vi "Set Exp Time.vi"(0 "Notifier Name":string, 7 "Exp Time (s)":dbl, 11 "Error In":errorcluster) -> (4 "Notifier Name DUP":string, 6 "Running?":bool, 10 "Image Ref":T1, 15 "Error Out":errorcluster)   [LabVIEW 2020]
uses:
  <vilib>/vision/Image Controls.llb/IMAQ Image.ctl
  Hardware Configuration/Hardware Configuration Controls/Company.ctl
  Hamamatsu/Orca Flash/Orca Flash Controls/Orca Flash Parameters.ctl
  Hamamatsu/Orca Flash/Orca Flash Controls/Orca Flash Parameter List.ctl
  Hamamatsu/Orca Flash/Orca Flash Controls/Orca Flash Actions.ctl
  IDS/IDS Controls/IDS Actions.ctl
  IDS/IDS Controls/IDS Parameters.ctl
  IDS/IDS Controls/IDS Parameter List.ctl
  Photometrics/Prime BSI/R Cubed SITK/Prime BSI R3 Controls/Prime R3 Actions.ctl
  Photometrics/Prime BSI/R Cubed SITK/Prime BSI R3 Controls/Prime R3 Parameters.ctl
  Photometrics/Prime BSI/R Cubed SITK/Prime BSI R3 Controls/Prime R3 Parameter List.ctl
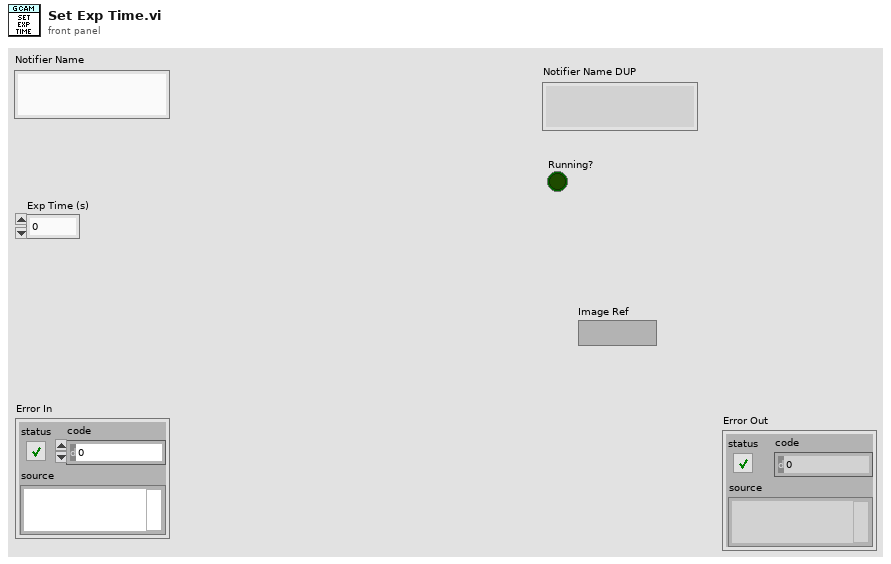
[diagram p1: front panel]
types:
  T1 = typedef "IMAQ Image.ctl" = refnum<image>
  T2 = typedef "Company.ctl" = enum16{"AA Opto Electronic", "ASI", "Coherent", "Creset Optics", "CVI", "DAQmx", "Hamamatsu", "IDS", "Mad City Labs", "Marzhauser", "Measurement Computing", "MPB Com", "Olympus", "Photometrics", "PI", "Prior", "Thorlabs"}
  T3 = typedef "Orca Flash Actions.ctl" = enum16{"Idle", "Preview", "Record", "Record Settings", "Set Param", "Get Param", "Set ROI", "Get ROI", "Trigger Source", "Trigger Type", "Progessive Mode", "Area Mode", "Status", "Quit"}
  T4 = typedef "Orca Flash Parameters.ctl" = cluster{"Value":dbl, "Parameter":T5}
  T5 = typedef "Orca Flash Parameter List.ctl" = u32
  T6 = typedef "IDS Parameter List.ctl" = enum16{"Exposure Time (s)", "Binning"}
  T7 = typedef "IDS Parameters.ctl" = cluster{"Parameter":T6, "Value":dbl}
  T8 = typedef "IDS Actions.ctl" = enum16{"Error Check", "Initialize", "Preview", "Record", "Abort", "Record Settings", "Set Parameter", "Get Parameter", "Set ROI", "Get ROI", "Status", "Quit"}
  T9 = typedef "Prime R3 Parameter List.ctl" = enum16{"Exposure Time (s)"}
  T10 = typedef "Prime R3 Parameters.ctl" = cluster{"Parameter":T9, "Value":dbl}
  T11 = typedef "Prime R3 Actions.ctl" = enum16{"Error Check", "Initialize", "Preview", "Record", "Abort", "Record Settings", "Set Parameter", "Get Parameter", "Set ROI", "Get ROI", "Status", "Set Trigger", "Quit"}
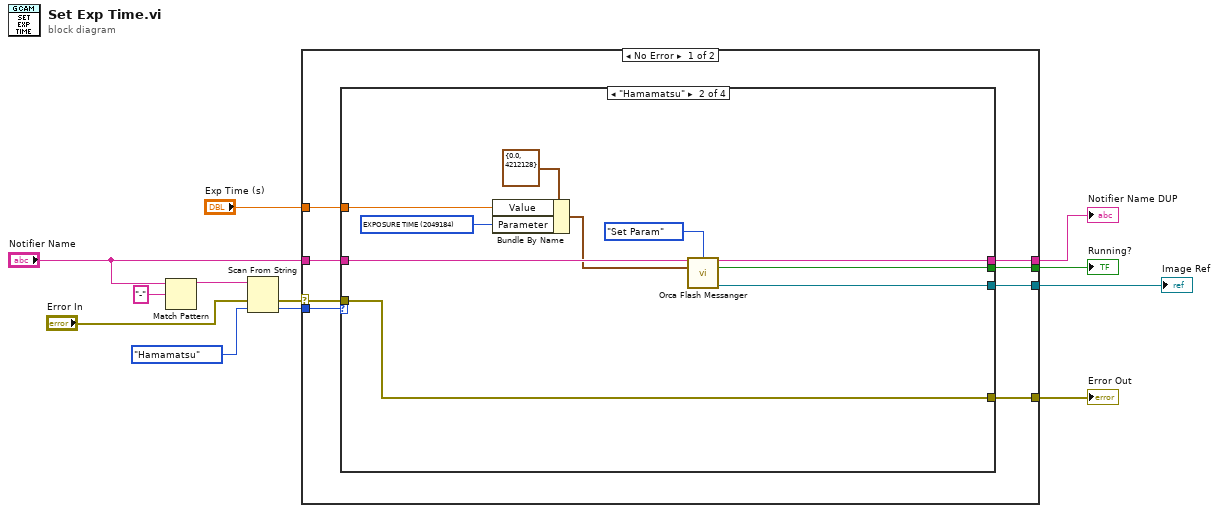
[diagram p0: block diagram]
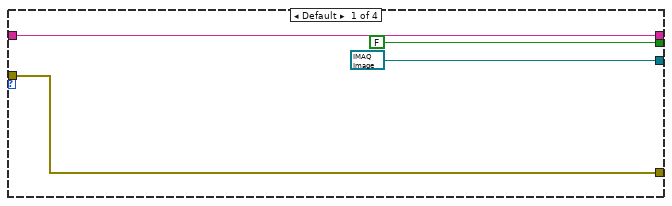
[diagram p2: hidden frame]
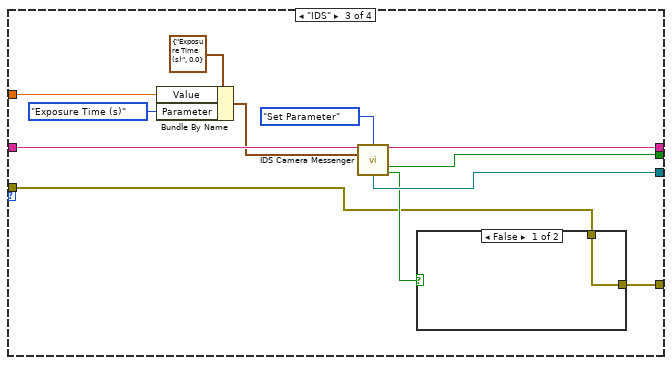
[diagram p3: hidden frame]
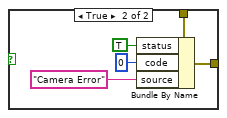
[diagram p4: hidden frame]
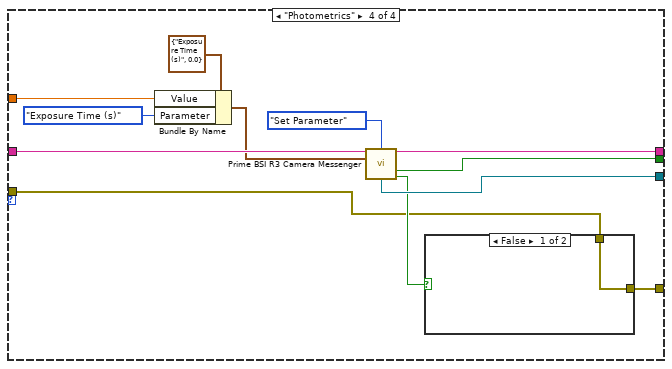
[diagram p5: hidden frame]
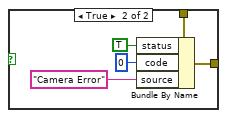
[diagram p6: hidden frame]
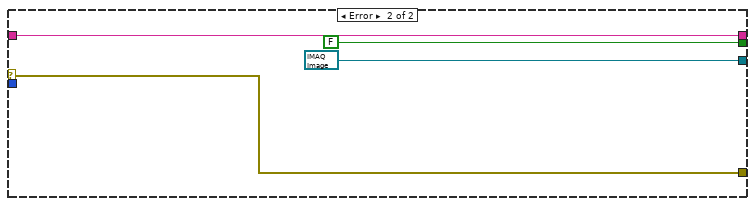
[diagram p7: hidden frame]
diagram:
  n1 = Match Pattern(string="Notifier Name", regular expression="-") -> (before substring=w10:string)  [unwired: 1 in, 3 out]
  n2 = Scan From String(input string=w10, error in="Error In", default 1=Company."Hamamatsu" ("Company")) -> (error out=w6:errorcluster, output 1=w9:T2)  [unwired: 2 in, 2 out]
  n3 = case shown="No Error" w6 {
    selector: w6 -> [w16 w73]
    tunnel: w9 -> [w20 _]
    tunnel: "Notifier Name" -> [w19 w74]
    tunnel: [w18 T1 refnum ("Image Ref")] -> w4
    tunnel: [w17 FALSE ("Running?")] -> w5
    tunnel: [w15 w74] -> w3
    tunnel: [w14 w73] -> w2
    tunnel: "Exp Time (s)" -> [w13 _]
    frame No Error {
      n4 = case shown="\"Hamamatsu\"" w20 {
        tunnel: w19 -> [w24 w34 w46 w64]
        tunnel: [T1 refnum ("Image Ref") w33 w44 w62] -> w18
        tunnel: [FALSE ("Running?") w32 w43 w61] -> w17
        tunnel: w16 -> [w23 w30 w40 w59]
        tunnel: [w24 w31 w45 w63] -> w15
        tunnel: [w23 w30 w39 w58] -> w14
        tunnel: w13 -> [_ w27 w37 w55]
        frame Default {
        }
        frame "Hamamatsu" {
          w29 = T5 2049184 items=["SENSOR MODE"=4212128, "READOUT SPEED"=4211872, "READOUT DIRECTION"=4211904, "TRIGGER GLOBAL EXPOSURE"=2049680, "TRIGGER DELAY"=1066480, "SYNC READOUT SYSTEM BLANK"=1066528, "SENSOR COOLER"=2115248, "SENSOR COOLER STATUS"=2115280, "EXPOSURE TIME"=2049184, "DEFECT CORRECT MODE"=4670368, "BINNING"=4215968, "INTERNAL LINE SPEED"=4226000, "INTERNAL LINE INTERVAL"=4226016, "IMAGE PIXEL TYPE"=4343296, "NUMBER OF OUTPUT TRIGGER CONNECTOR"=1852320, "OUTPUT TRIGGER SOURCE[0]"=1852576, "OUTPUT TRIGGER SOURCE[1]"=1852832, "OUTPUT TRIGGER SOURCE[2]"=1853088, "OUTPUT TRIGGER POLARITY[0]"=1852592, "OUTPUT TRIGGER POLARITY[1]"=1852848, "OUTPUT TRIGGER POLARITY[2]"=1853104, "OUTPUT TRIGGER ACTIVE[0]"=1852608, "OUTPUT TRIGGER ACTIVE[1]"=1852864, "OUTPUT TRIGGER ACTIVE[2]"=1853120, "OUTPUT TRIGGER DELAY[0]"=1852624, "OUTPUT TRIGGER DELAY[1]"=1852880, "OUTPUT TRIGGER DELAY[2]"=1853136, "OUTPUT TRIGGER PERIOD[0]"=1852640, "OUTPUT TRIGGER PERIOD[1]"=1852896, "OUTPUT TRIGGER PERIOD[2]"=1853152, "OUTPUT TRIGGER KIND[0]"=1852656, "OUTPUT TRIGGER KIND[1]"=1852912, "OUTPUT TRIGGER KIND[2]"=1853168, "OUTPUT TRIGGER PRE HSYNC COUNT"=1852704] ("Parameter")
          n5 = Bundle By Name(cluster=T4 {"Value"=0.0, "Parameter"=4212128} ("sCMOS Parameter"), "Value"=w27, "Parameter"=w29) -> (w26:T4)
          n6 = call "Orca Flash Messanger.vi"("Notifier Name"=w34, "Camera Actions"=Orca_Flash_Actions."Set Param", "sCMOS Parameter"=w26) -> ("Notifier Name Dup"=w31:string, "Running?"=w32:bool, "Image Ref"=w33:T1)  [unwired: 8 in, 2 out]
        }
        frame "IDS" {
          n7 = Bundle By Name(cluster=T7 {"Parameter"=enum."Exposure Time (s)", "Value"=0.0} ("IDS Parameter"), "Value"=w37, "Parameter"=IDS_Parameter_List."Exposure Time (s)") -> (w35:T7)
          n8 = call "IDS Camera Messenger.vi"("Notifier Name"=w46, "IDS Actions"=IDS_Actions."Set Parameter", "IDS Parameter"=w35) -> ("Notifier Name (Dup)"=w45:string, "Running?"=w43:bool, "Image Ref"=w44:T1, "Error?"=w41:bool)  [unwired: 7 in, 2 out]
          n9 = case shown="False" w41 {
            tunnel: w40 -> [w47 w52]
            tunnel: [w47 w51] -> w39
            frame False {
            }
            frame True {
              n10 = Bundle By Name(cluster=w52, "status"=TRUE, "code"=0, "source"="Camera Error") -> (w51:errorcluster)
            }
          }
        }
        frame "Photometrics" {
          n11 = Bundle By Name(cluster=T10 {"Parameter"=enum."Exposure Time (s)", "Value"=0.0} ("Prime Parameter"), "Value"=w55, "Parameter"=Prime_R3_Parameter_List."Exposure Time (s)") -> (w53:T10)
          n12 = call "Prime BSI R3 Camera Messenger.vi"("Notifier Name"=w64, "Prime Actions"=Prime_R3_Actions."Set Parameter", "Prime Parameter"=w53) -> ("Notifier Name (Dup)"=w63:string, "Running?"=w61:bool, "Image Ref"=w62:T1, "Error?"=w60:bool)  [unwired: 7 in, 2 out]
          n13 = case shown="False" w60 {
            tunnel: w59 -> [w65 w70]
            tunnel: [w65 w69] -> w58
            frame False {
            }
            frame True {
              n14 = Bundle By Name(cluster=w70, "status"=TRUE, "code"=0, "source"="Camera Error") -> (w69:errorcluster)
            }
          }
        }
      }
    }
    frame Error {
    }
  }
  "Error Out" <- w2
  "Notifier Name DUP" <- w3
  "Image Ref" <- w4
  "Running?" <- w5
